vi "Middle_ILA_use.vi"() -> ()   [LabVIEW 2017]
panel:
  in  "address":string="10.3.173.11"
  in  "error in (no error)":errorcluster
  out "error out":errorcluster
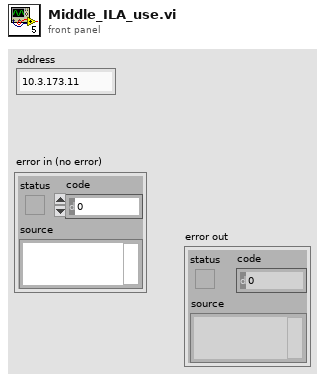
[diagram p1: front panel]
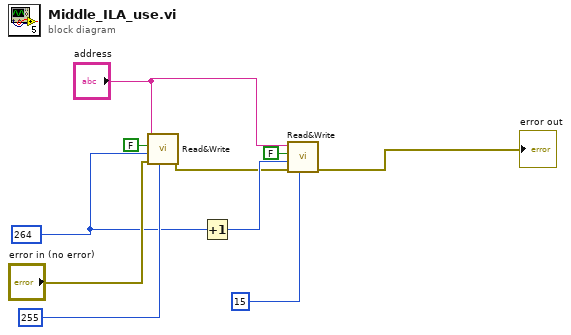
[diagram p0: block diagram]
diagram:
  w5 = u32 264 ("Address")
  n1 = call "Read&Write.vi"("In"=u8 255, "error in (no error)"="error in (no error)", "Address"=w5, "Read (TRUE)"=FALSE, "address"="address") -> ("error out"=w2:errorcluster)  [unwired: 5 in, 1 out]
  n2 = Increment(x=w5) -> (x+1=w6:u32)
  n3 = call "Read&Write.vi"("In"=u8 15, "error in (no error)"=w2, "Address"=w6, "Read (TRUE)"=FALSE, "address"="address") -> ("error out"=→"error out":errorcluster)  [unwired: 5 in, 1 out]
